vi "PathPlanner_Path_WaypointsFromPoses.vi"(11 "Poses":T3[](array[typedef]) {"ROTATION"."SIN" format="%13.4f"; "ROTATION"."COS" format="%13.4f"; "ROTATION"."VALUE" format="%13.4f"; "TRANSLATION"."Y" format="%14.3f"; "TRANSLATION"."X" format="%14.3f"}) -> (0 "Error":bool, 3 "Waypoints":T1[](array[typedef]) {"nextControl"."Y" format="%14.3f"; "nextControl"."X" format="%14.3f"; "anchor"."Y" format="%14.3f"; "anchor"."X" format="%14.3f"; "prevControl"."Y" format="%14.3f"; "prevControl"."X" format="%14.3f"})   [LabVIEW 2019, in "PathPlanner24.lvlib"]
doc: "Create the bezier points necessary to create a path using a list of poses\n\nInputs: \n - poses - pose2d array - List of poses. Each pose represents one waypoint.\n\nOutputs:\n - Waypoints - cluster array - Bezier curve waypoints\n - Error - boolean - TRUE if an error occured. (Too few poses)"
uses:
  PathPlanner24.lvlib
  <vilib>/Rock Robotics/WPI/ThirdParty/JAS_Junk/TrajLib/TypeDef/POSE2D.ctl
  <vilib>/Rock Robotics/WPI/ThirdParty/JAS_Junk/TrajLib/TypeDef/TRANSLATION2D.ctl
  <vilib>/Rock Robotics/WPI/ThirdParty/JAS_Junk/TrajLib/TypeDef/ROTATION2D.ctl
  TypeDef/PathPlannerWaypoint.ctl
  <vilib>/Rock Robotics/WPI/ThirdParty/JAS_Junk/TrajLib/Translation2d_Minus.vi
  <vilib>/Rock Robotics/WPI/ThirdParty/JAS_Junk/TrajLib/Translation2d_Create_DistAng.vi
  <vilib>/Rock Robotics/WPI/ThirdParty/JAS_Junk/TrajLib/Translation2d_GetDistance.vi
  PathPlanner_Waypoint_AutoCtrlDistFactor.vi
  <vilib>/Rock Robotics/WPI/ThirdParty/JAS_Junk/TrajLib/Translation2d_Plus.vi
  <vilib>/Rock Robotics/WPI/ThirdParty/JAS_Junk/TrajLib/Translation2d_Create.vi
  <vilib>/Rock Robotics/WPI/ThirdParty/JAS_Junk/TrajLib/Rotation2d_GetAngleCosSin.vi
  <vilib>/Rock Robotics/WPI/ThirdParty/JAS_Junk/TrajLib/Util_CalcDist.vi
  <vilib>/Rock Robotics/WPI/ThirdParty/JAS_Junk/TrajLib/Trajectory_Library.lvlib
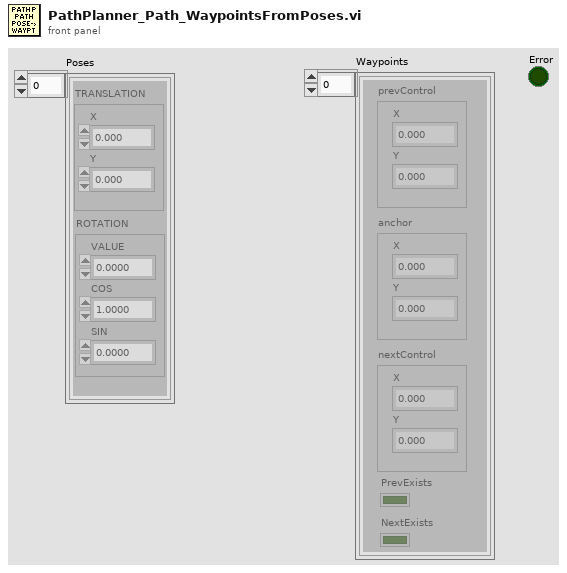
[diagram p1: front panel]
types:
  T1 = typedef "PathPlanner24.lvlib/PathPlannerWaypoint.ctl" = cluster{"prevControl":T2, "anchor":T2, "nextControl":T2, "PrevExists":bool, "NextExists":bool}
  T2 = typedef "Trajectory_Library.lvlib/TRANSLATION2D.ctl" = cluster{"X":dbl, "Y":dbl}
  T3 = typedef "Trajectory_Library.lvlib/POSE2D.ctl" = cluster{"TRANSLATION":T2, "ROTATION":T4}
  T4 = typedef "Trajectory_Library.lvlib/ROTATION2D.ctl" = cluster{"VALUE":dbl, "COS":dbl, "SIN":dbl}
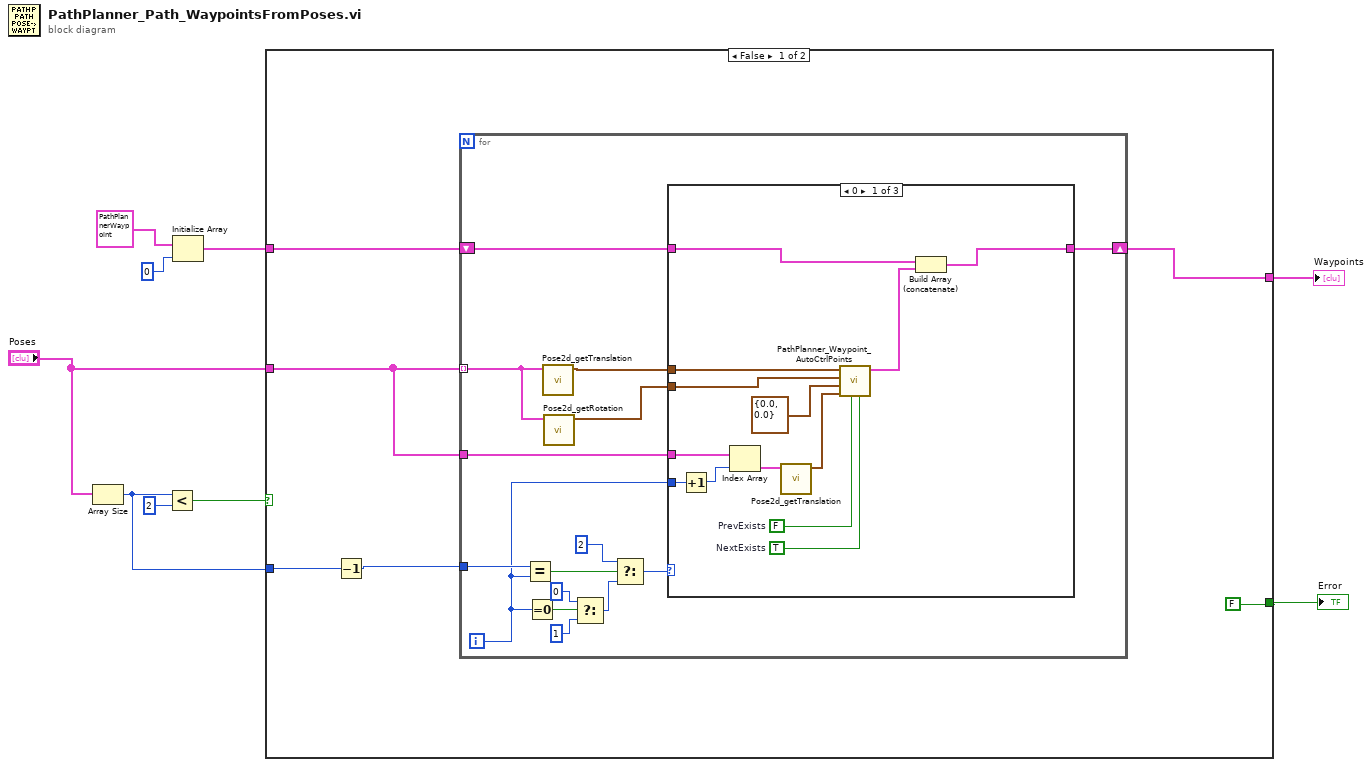
[diagram p0: block diagram]
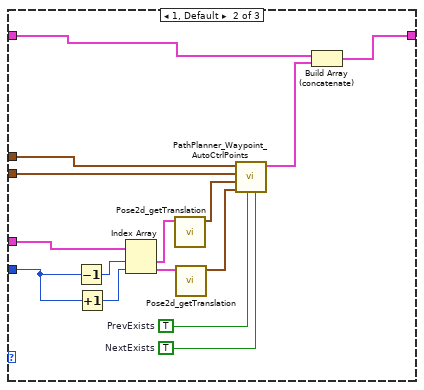
[diagram p2: hidden frame]
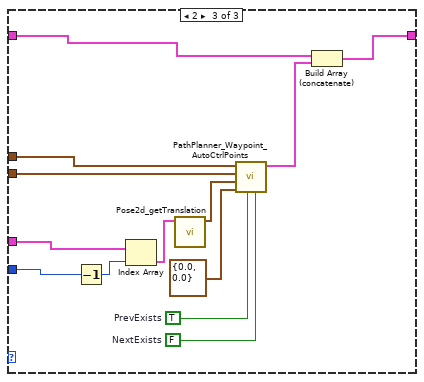
[diagram p3: hidden frame]
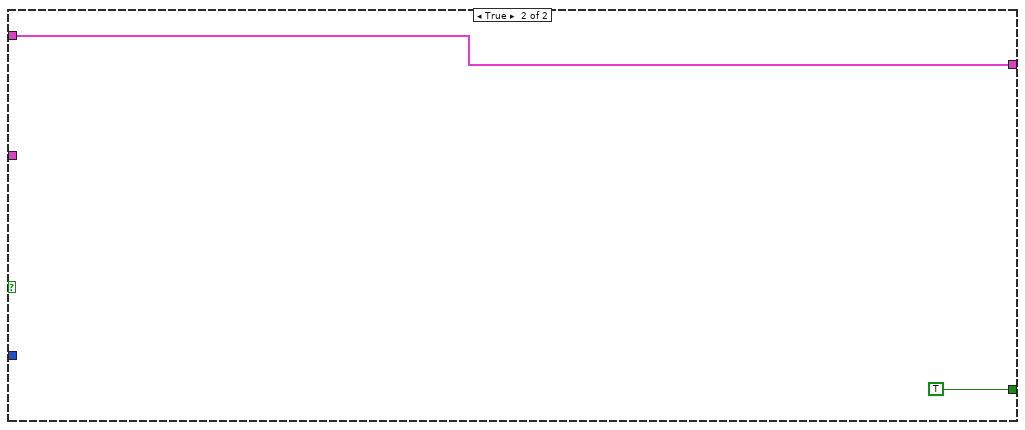
[diagram p4: hidden frame]
diagram:
  n1 = Array Size(array="Poses") -> (size(s)=w1:i32)
  n2 = Less?(x=w1, y=2) -> (x < y?=w6:bool)
  n3 = Initialize Array(T1 {"prevControl"={"X"=0.0, "Y"=0.0}, "anchor"={"X"=0.0, "Y"=0.0}, "nextControl"={"X"=0.0, "Y"=0.0}, "PrevExists"=FALSE, "NextExists"=FALSE} ("Bezier"), 0 ("dimension size")) -> (w5:T1[])
  n4 = case shown="False" w6 {
    tunnel: w5 -> [w14 w72]
    tunnel: [w10 w72] -> w2
    tunnel: [FALSE TRUE] -> w4
    tunnel: "Poses" -> [w11 _]
    tunnel: w1 -> [w12 _]
    frame False {
      n5 = Decrement(x=w12) -> (x-1=w13:i32)
      n6 = for {
        tunnel: w11 -> [w22] mode=indexing
        shift-right: [w16] -> w10
        shift-left: w14 -> [w17]
        tunnel: w13 -> [w30]
        tunnel: w11 -> [w19]
        i -> [w18]
        n7 = Equal?(x=w30, y=w18) -> (x = y?=w24:bool)
        n8 = Equal To 0?(x=w18) -> (x = 0?=w29:bool)
        n9 = call <vilib>:"Pose2d_getTranslation.vi"("in POSE"=w22) -> ("outTRANSLATION"=w21:T2)  [unwired: 10 in]
        n10 = call <vilib>:"Pose2d_getRotation.vi"("in POSE"=w22) -> ("out ROTATION"=w20:T4)  [unwired: 10 in]
        n11 = Select(t=i16 0 ("f"), s=w29, f=i16 1) -> (s? t:f=w26:i16)
        n12 = Select(t=i16 2 ("f"), s=w24, f=w26) -> (s? t:f=w23:i16)
        n13 = case shown="0" w23 {
          tunnel: w21 -> [w43 w49 w65]
          tunnel: w20 -> [w42 w48 w64]
          tunnel: w19 -> [w41 w53 w68]
          tunnel: w18 -> [w40 w55 w70]
          tunnel: w17 -> [w36 w47 w63]
          tunnel: [w34 w46 w62] -> w16
          frame 0 {
            w32 = TRUE  # NextExists
            w33 = FALSE  # PrevExists
            n14 = Increment(x=w40) -> (x+1=w39:i32)
            n15 = Index Array(array=w41, index=w39) -> (element=w38:T3)
            n16 = call <vilib>:"Pose2d_getTranslation.vi"("in POSE"=w38) -> ("outTRANSLATION"=w37:T2)  [unwired: 10 in]
            n17 = call "PathPlanner_Waypoint_AutoCtrlPoints.vi"("NextExists"=w32, "PrevExists"=w33, "NextAnchor"=w37, "PrevAnchor"=T2 {"X"=0.0, "Y"=0.0} ("NextAnchor"), "Heading"=w42, "Anchor"=w43) -> ("Waypoint"=w35:T1)  [unwired: 5 in]
            n18 = Build Array (concatenate)(w36, w35) -> (w34:T1[])
          }
          frame 1, Default {
            w44 = TRUE  # NextExists
            w45 = TRUE  # PrevExists
            n19 = Decrement(x=w55) -> (x-1=w54:i32)
            n20 = Increment(x=w55) -> (x+1=w56:i32)
            n21 = Index Array(array=w53, index #1=w54, index #2=w56) -> (element #1=w50:T3, element #2=w51:T3)
            n22 = call <vilib>:"Pose2d_getTranslation.vi"("in POSE"=w50) -> ("outTRANSLATION"=w52:T2)  [unwired: 10 in]
            n23 = call <vilib>:"Pose2d_getTranslation.vi"("in POSE"=w51) -> ("outTRANSLATION"=w58:T2)  [unwired: 10 in]
            n24 = call "PathPlanner_Waypoint_AutoCtrlPoints.vi"("NextExists"=w44, "PrevExists"=w45, "NextAnchor"=w58, "PrevAnchor"=w52, "Heading"=w48, "Anchor"=w49) -> ("Waypoint"=w57:T1)  [unwired: 5 in]
            n25 = Build Array (concatenate)(w47, w57) -> (w46:T1[])
          }
          frame 2 {
            w60 = FALSE  # NextExists
            w61 = TRUE  # PrevExists
            n26 = Decrement(x=w70) -> (x-1=w69:i32)
            n27 = Index Array(array=w68, index=w69) -> (element=w66:T3)
            n28 = call <vilib>:"Pose2d_getTranslation.vi"("in POSE"=w66) -> ("outTRANSLATION"=w67:T2)  [unwired: 10 in]
            n29 = call "PathPlanner_Waypoint_AutoCtrlPoints.vi"("NextExists"=w60, "PrevExists"=w61, "NextAnchor"=T2 {"X"=0.0, "Y"=0.0}, "PrevAnchor"=w67, "Heading"=w64, "Anchor"=w65) -> ("Waypoint"=w71:T1)  [unwired: 5 in]
            n30 = Build Array (concatenate)(w63, w71) -> (w62:T1[])
          }
        }
      }
    }
    frame True {
    }
  }
  "Waypoints" <- w2
  "Error" <- w4
